vi "CreateTargetDoseNode.vi"(8 "Error In":errorcluster, 10 "Experiment":T1={"File Path"=path "", "Operator"="Operator", "Project"="Project Description", "Target Dose (dpa)"=0.0, "Sample"={"Name"="", "Description"="", "Molar Mass (g/mol)"=0.0, "Density (g/cm^3)"=0.0, "Irradiation Area (cm^2)"=0.0, "SRIM Damage Peak (disp * ions/cm)"=0.0}, "Beam Line"={"Type"=enum."Ion Beam Analysis", "Ion"=enum."H", "Charge State"=0, "Total Source Ion Energy (kV)"=nan}, "Runs"=[]} {"Beam Line"."Charge State" min=1}, 11 "DOM Document In":refnum<k20>) -> (0 "Error out":errorcluster, 2 "Target Dose Node":refnum<k20>, 3 "DOM Document Out":refnum<k20>)   [LabVIEW 2012]
uses:
  Experiment.ctl
  Sample.ctl
  BeamLine.ctl
  BeamLineType.ctl
  BeamLineIon.ctl
  ExperimentRun.ctl
  ExperimentRunTiming.ctl
  ExperimentRunDose.ctl
  ExperimentRunFluence.ctl
  ExperimentRunTotalCharge.ctl
  <resource>/objmgr/DOMUserDefRef.rc
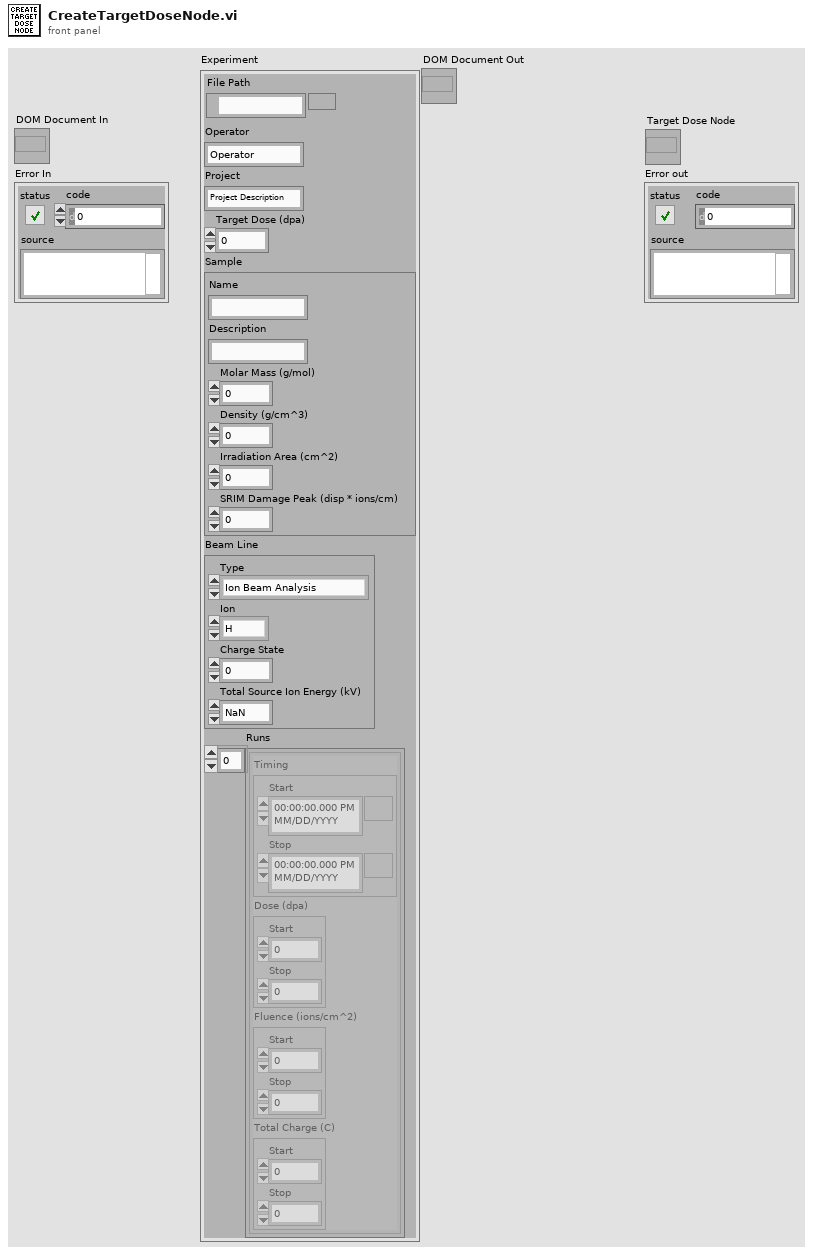
[diagram p1: front panel]
types:
  T1 = typedef "Experiment.ctl" = cluster{"File Path":path, "Operator":string, "Project":string, "Target Dose (dpa)":dbl, "Sample":T2, "Beam Line":T3, "Runs":T6[]}
  T2 = typedef "Sample.ctl" = cluster{"Name":string, "Description":string, "Molar Mass (g/mol)":dbl, "Density (g/cm^3)":dbl, "Irradiation Area (cm^2)":dbl, "SRIM Damage Peak (disp * ions/cm)":dbl}
  T3 = typedef "BeamLine.ctl" = cluster{"Type":T4, "Ion":T5, "Charge State":u8, "Total Source Ion Energy (kV)":dbl}
  T4 = typedef "BeamLineType.ctl" = enum16{"Ion Beam Analysis", "Auxiliary", "Radiation Damage"}
  T5 = typedef "BeamLineIon.ctl" = enum16{"H", "He", "C", "Fe", "Ni", "Pt", "Si", "Ag", "Au"}
  T6 = typedef "ExperimentRun.ctl" = cluster{"Timing":T7, "Dose (dpa)":T8, "Fluence (ions/cm^2)":T9, "Total Charge (C)":T10}
  T7 = typedef "ExperimentRunTiming.ctl" = cluster{"Start":timestamp, "Stop":timestamp}
  T8 = typedef "ExperimentRunDose.ctl" = cluster{"Start":dbl, "Stop":dbl}
  T9 = typedef "ExperimentRunFluence.ctl" = cluster{"Start":dbl, "Stop":dbl}
  T10 = typedef "ExperimentRunTotalCharge.ctl" = cluster{"Start":dbl, "Stop":dbl}
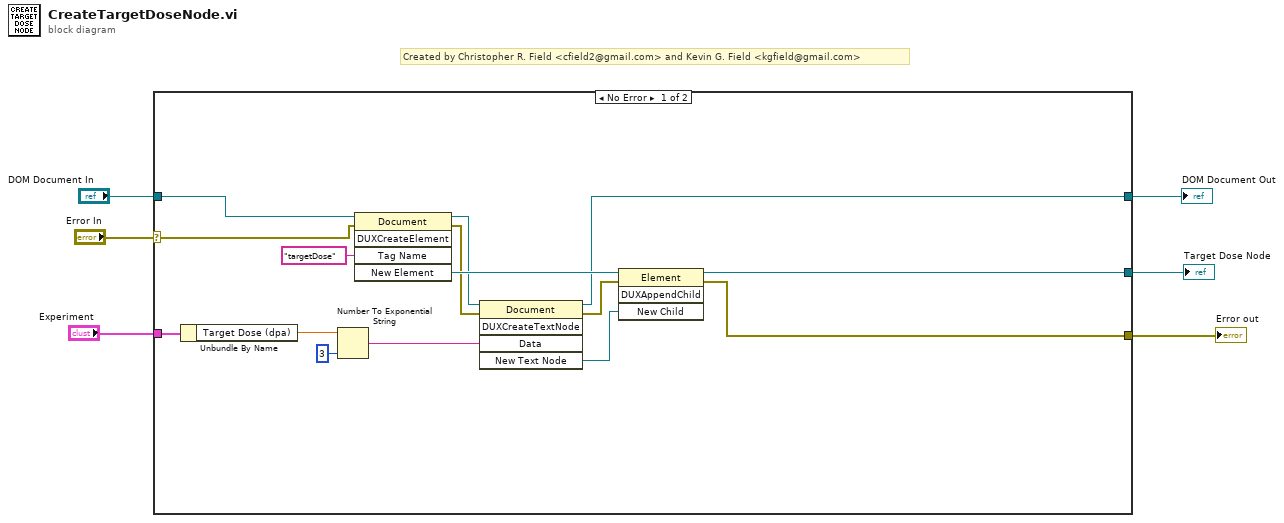
[diagram p0: block diagram]
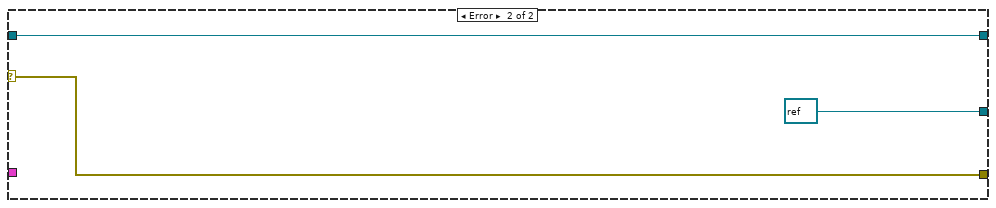
[diagram p2: hidden frame]
diagram:
  # "Created by Christopher R. Field <cfield2@gmail.com> and Kevin G. Field <kgfield@gmail.com>"
  n1 = case shown="No Error" "Error In" {
    selector: "Error In" -> [w11 w23]
    tunnel: "DOM Document In" -> [w21 w24]
    tunnel: [w20 refnum<k20> refnum ("Operator Node 2")] -> w5
    tunnel: [w19 w23] -> w4
    tunnel: "Experiment" -> [w12 _]
    tunnel: [w10 w24] -> w1
    frame No Error {
      n2 = Unbundle By Name(w12) -> ("Target Dose (dpa)"=w9:dbl)
      n3 = Number To Exponential String(number=w9, precision (6)=i16 3) -> (E-format string=w8:string)  [unwired: 2 in]
      n4 = invoke class="Document" method="DUXCreateElement"(reference=w21, error in=w11, "Tag Name"="targetDose") -> (reference out=w16:refnum<k20>, error out=w15:errorcluster, "New Element"=w17:refnum<k20>)  [unwired: 2 in, 2 out]
      n5 = invoke class="Document" method="DUXCreateTextNode"(reference=w16, error in=w15, "Data"=w8) -> (reference out=w10:refnum<k20>, error out=w14:errorcluster, "New Text Node"=w13:refnum<k20>)  [unwired: 2 in, 2 out]
      n6 = invoke class="Element" method="DUXAppendChild"(reference=w17, error in=w14, "New Child"=w13) -> (reference out=w20:refnum<k20>, error out=w19:errorcluster)  [unwired: 1 in, 2 out]
    }
    frame Error {
    }
  }
  "Target Dose Node" <- w5
  "Error out" <- w4
  "DOM Document Out" <- w1
